vi "Create Segment Velocities.vi"(9 "Conditions":T1, 10 "Velocities":dbl[](array[numeric]), 11 "upper limit":T2) -> (3 "Velocities":dbl[](array[numeric]))   [LabVIEW 2019]
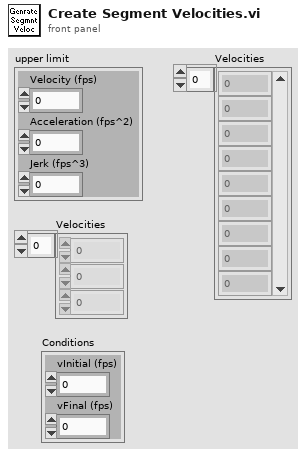
[diagram p1: front panel]
types:
  T1 = cluster{"vInitial (fps)":dbl, "vFinal (fps)":dbl}
  T2 = cluster{"Velocity (fps)":dbl, "Acceleration (fps^2)":dbl, "Jerk (fps^3)":dbl}
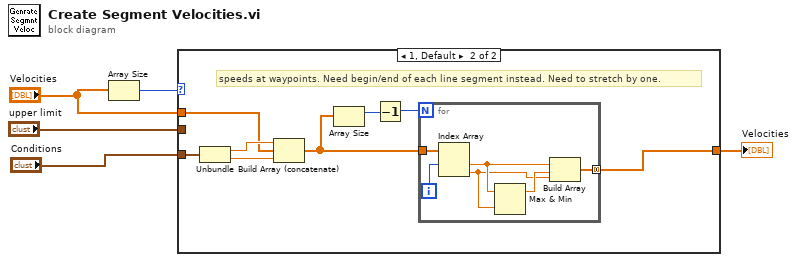
[diagram p0: block diagram]
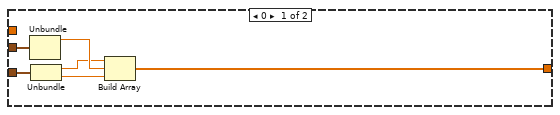
[diagram p2: hidden frame]
diagram:
  n1 = Array Size(array="Velocities") -> (size(s)=w1:i32)
  n2 = case shown="1, Default" w1 {
    tunnel: "Conditions" -> [w11 w17]
    tunnel: "Velocities" -> [_ w16]
    tunnel: "upper limit" -> [w10 _]
    tunnel: [w6 w12] -> w5
    frame 0 {
      n3 = Unbundle(w10) -> ("Velocity (fps)"=w9:dbl)  [unwired: 2 out]
      n4 = Unbundle(w11) -> ("vInitial (fps)"=w8:dbl, "vFinal (fps)"=w7:dbl)
      n5 = Build Array(w8, w9, w7) -> (w6:dbl[])
    }
    frame 1, Default {
      # "speeds at waypoints. Need begin/end of each line segment instead. Need to stretch by one."
      n6 = Unbundle(w17) -> ("vInitial (fps)"=w19:dbl, "vFinal (fps)"=w18:dbl)
      n7 = Build Array (concatenate)(w19, w16, w18) -> (w13:dbl[])
      n8 = Array Size(array=w13) -> (size(s)=w14:i32)
      n9 = Decrement(x=w14) -> (x-1=w15:i32)
      n10 = for {
        N: w15 -> [_]
        tunnel: w13 -> [w25]
        tunnel: [w20] -> w12 mode=concatenating
        i -> [w24]
        n11 = Index Array(array=w25, index #1=w24) -> (element #1=w23:dbl, element #2=w21:dbl)  [unwired: 1 in]
        n12 = Max & Min(x=w23, y=w21) -> (max(x,y)=w22:dbl)  [unwired: 1 out]
        n13 = Build Array(w23, w22, w21) -> (w20:dbl[])
      }
    }
  }
  "Velocities" <- w5
